vi "getTime.vi"() -> (0 "시간":string, 3 "날짜":string)   [LabVIEW 2010]
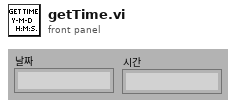
[diagram p1: front panel]
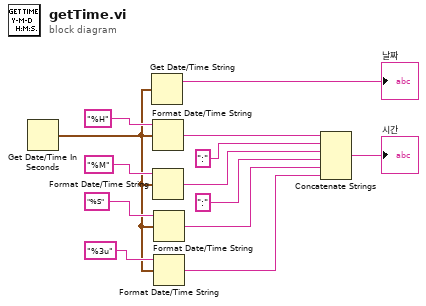
[diagram p0: block diagram]
diagram:
  n1 = Get Date/Time In Seconds() -> (seconds since 1Jan1904=w2:timestamp)
  n2 = Get Date/Time String(seconds (now)=w2) -> (date string=→"날짜":string)  [unwired: 2 in, 1 out]
  n3 = Format Date/Time String(time format string (%c)="%H" ("시간 포맷 문자열 (%c)"), seconds (now)=w2) -> (date/time string=w9:string)  [unwired: 1 in]
  n4 = Format Date/Time String(time format string (%c)="%M" ("시간 포맷 문자열 (%c)"), seconds (now)=w2) -> (date/time string=w8:string)  [unwired: 1 in]
  n5 = Format Date/Time String(time format string (%c)="%S" ("시간 포맷 문자열 (%c)"), seconds (now)=w2) -> (date/time string=w6:string)  [unwired: 1 in]
  n6 = Format Date/Time String(time format string (%c)="%3u" ("시간 포맷 문자열 (%c)"), seconds (now)=w2) -> (date/time string=w1:string)  [unwired: 1 in]
  n7 = Concatenate Strings(w9, ":" ("문자열"), w8, ":" ("문자열"), w6, w1) -> (→"시간":string)
